vi "Make API Call From Control.vi"() -> ()   [LabVIEW 2018, in "Scripting.lvlib"]
uses:
  Scripting.lvlib
panel:
  out "error out 2":errorcluster
  in  "error in (no error)":errorcluster
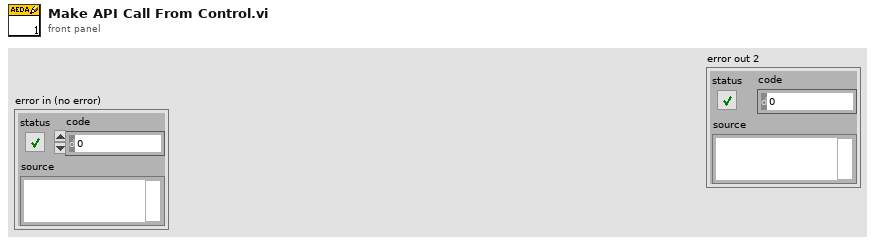
[diagram p1: front panel]
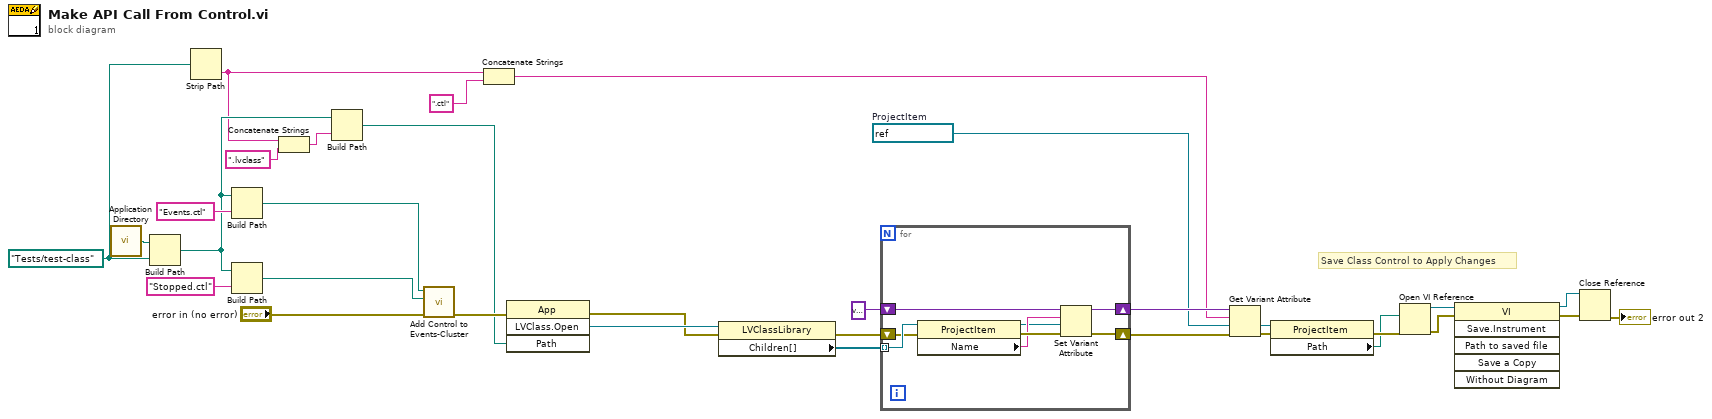
[diagram p0: block diagram]
diagram:
  w10 = refnum<vi> refnum  # ProjectItem
  w16 = path "Tests/test-class" ("Typedef:Path")
  # "Save Class Control to Apply Changes"
  n1 = call <vilib>:"Application Directory.vi"() -> ("Application Directory"=w32:path)
  n2 = Build Path(base path=w32, name or relative path=w16) -> (appended path=w25:path)
  n3 = Strip Path(path=w16) -> (name=w12:string)  [unwired: 1 out]
  n4 = Build Path(base path=w25, name or relative path="Events.ctl") -> (appended path=w28:path)
  n5 = Build Path(base path=w25, name or relative path="Stopped.ctl") -> (appended path=w27:path)
  n6 = Concatenate Strings(w12, ".lvclass" ("string")) -> (w11:string)
  n7 = Build Path(base path=w25, name or relative path=w11) -> (appended path=w24:path)
  n8 = call "Add Control to Events-Cluster.vi"("error in (no error)"="error in (no error)", "Control to Add"=w27, "Events Type-Def Path"=w28) -> ("error out"=w26:errorcluster)  [unwired: 8 in]
  n9 = Concatenate Strings(w12, ".ctl" ("string")) -> (w15:string)
  n10 = invoke class="App" method="LVClass.Open"(error in=w26, "Path"=w24) -> (error out=w22:errorcluster, "LVClass.Open"=w23:refnum<vi>)  [unwired: 2 in, 2 out]
  n11 = property class="LVClassLibrary"(reference=w23, error in=w22) -> (error out=w20:errorcluster, "Children[]"=w21:refnum<vi>[])  [unwired: 1 out]
  n12 = for {
    tunnel: w21 -> [w40] mode=indexing
    shift-right: [w34] -> w17
    shift-left: w20 -> [w39]
    shift-right: [w35] -> w18
    shift-left: variant ("variant") -> [w36]
    n13 = property class="ProjectItem"(reference=w40, error in=w39) -> (reference out=w33:refnum<vi>, error out=w38:errorcluster, "Name"=w37:string)
    n14 = Set Variant Attribute(Variant=w36, name=w37, value=w33, error in=w38) -> (Variant out=w35:variant, error out=w34:errorcluster)  [unwired: 1 out]
  }
  n15 = Get Variant Attribute(Variant=w18, name=w15, default value (empty Variant)=w10, error in=w17) -> (value=w9:refnum<vi>, error out=w8:errorcluster)  [unwired: 2 out]
  n16 = property class="ProjectItem"(reference=w9, error in=w8) -> (error out=w7:errorcluster, "Path"=w6:path)  [unwired: 1 out]
  n17 = Open VI Reference(vi path=w6, error in (no error)=w7) -> (vi reference=w5:refnum<vi>, error out=w4:errorcluster)  [unwired: 4 in]
  n18 = invoke class="VI" method="Save.Instrument"(reference=w5, error in=w4) -> (reference out=w2:refnum<vi>, error out=w3:errorcluster)  [unwired: 4 in, 4 out]
  n19 = Close Reference(reference=w2, error in (no error)=w3) -> (error out=→"error out 2":errorcluster)
